vi "Untitled 3.vi"() -> ()   [LabVIEW 2019]
panel:
  out "output cluster":cluster{dbl, dbl}
  out "x/y":dbl
  out "Point out":cluster{"x":sgl, "y":sgl}
  out "x*y 2":dbl
  out "x*y":dbl
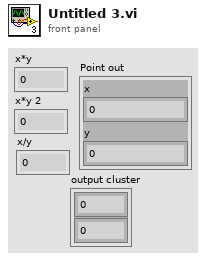
[diagram p1: front panel]
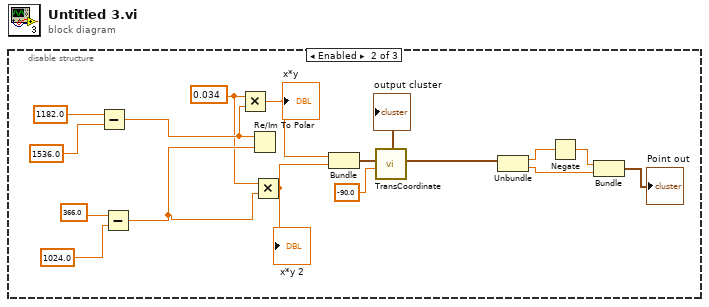
[diagram p0: block diagram]
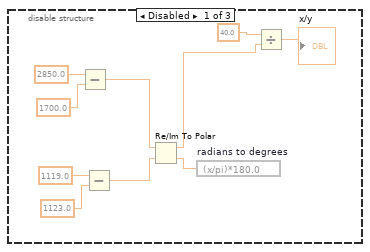
[diagram p2: hidden frame]
diagram:
  n1 = disable-structure shown="Enabled" {
    frame Disabled {
      n2 = Subtract(x=2850.0, y=1700.0 ("x")) -> (x-y=w6:dbl)
      n3 = Subtract(x=1119.0, y=1123.0 ("x")) -> (x-y=w5:dbl)
      n4 = Re/Im To Polar(2:w5, 3:w6) -> (0:w4:dbl, 1:w2:dbl)
      n5 = expression code="(x/pi)*180.0" "radians to degrees"(w4) -> ()  [unwired: 1 out]
      n6 = Divide(x=40.0, y=w2) -> (x/y=→"x/y":dbl)
    }
    frame Enabled {
      w11 = 0.034 ("x/y")
      n7 = Subtract(x=1182.0, y=1536.0) -> (x-y=w22:dbl)
      n8 = Subtract(x=366.0, y=1024.0) -> (x-y=w21:dbl)
      n9 = Multiply(x=w11, y=w22) -> (x*y=w19:dbl)
      "x*y" <- w19
      n10 = Re/Im To Polar(2:w21, 3:w22) -> ()  [unwired: 2 out]
      n11 = Multiply(x=w11, y=w21) -> (x*y=w18:dbl)
      "x*y 2" <- w18
      n12 = Bundle(w19, w18) -> (w20:cluster{dbl, dbl})  [unwired: 1 in]
      "output cluster" <- w20
      n13 = call "TransCoordinate.vi"("A"=sgl -90.0, "Point in"=w20) -> ("Point out"=w16:cluster{"x":sgl, "y":sgl})  [unwired: 9 in]
      n14 = Unbundle(w16) -> ("x"=w15:sgl, "y"=w13:sgl)
      n15 = Negate(x=w15) -> (-x=w14:sgl)
      n16 = Bundle(w14, "y"=w13) -> (→"Point out":cluster{sgl, "y":sgl})  [unwired: 1 in]
    }
    frame Disabled {
    }
  }
